vi "LevMar - abx.vi"(0 "Y":dbl[](array[numeric]) format="%0.2f", 1 "Target function in":refnum<vi>, 2 "Coefficients":dbl[](array[numeric]) format="%0.2f", 3 "Standard Deviation":dbl[](array[numeric]) caption="Écart-type" format="%0.2f") -> (5 "Target function out":refnum<vi>, 6 "Alpha":dbl[][](array[numeric]) format="%0.2f", 7 "Beta":dbl[](array[numeric]) caption="Bêta" format="%0.2f", 9 "chiSqr":dbl caption="khiCarré" format="%0.2f")   [LabVIEW 2009]
panel:
  # "Lev-Mar\nabx"
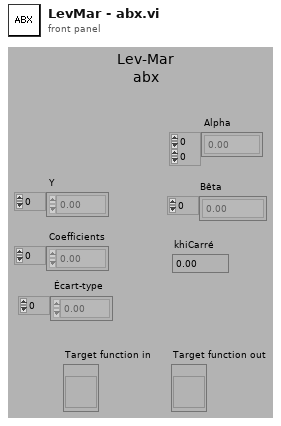
[diagram p1: front panel]
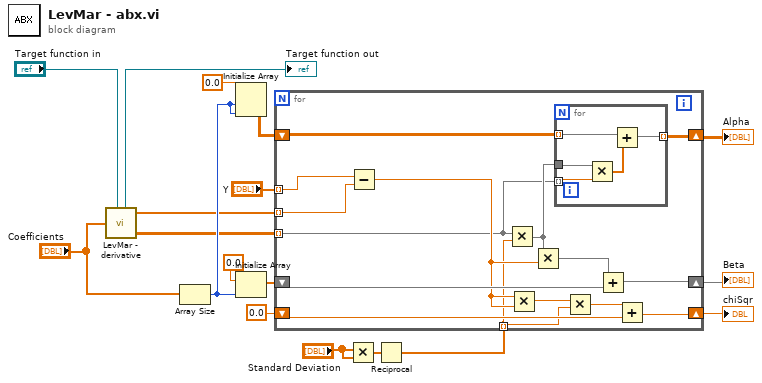
[diagram p0: block diagram]
diagram:
  n1 = call "LevMar - derivative.vi"("Target Function in"="Target function in", "Coefficients"="Coefficients") -> ("Target Function out"=→"Target function out":refnum<vi>, "F"=w2:dbl[], "dF/dA"=w4:dbl[][])  [unwired: 5 in]
  n2 = Array Size(array="Coefficients") -> (size(s)=w17:i32)
  n3 = Initialize Array(0.0, w17, w17) -> (w15:dbl[][])
  n4 = Initialize Array(0.0, w17) -> (w16:dbl[])
  n5 = Multiply(x="Standard Deviation", y="Standard Deviation") -> (x*y=w8:dbl[])
  n6 = Reciprocal(x=w8) -> (1/x=w6:dbl[])
  n7 = for {
    shift-right: [w29] -> w13
    shift-left: w16 -> [w30]
    shift-right: [w26] -> w10
    shift-left: w15 -> [w27]
    shift-right: [w25] -> w7
    shift-left: 0.0 -> [w32]
    tunnel: "Y" -> [w31] mode=indexing
    tunnel: w6 -> [w22] mode=indexing
    tunnel: w4 -> [w21] mode=indexing
    tunnel: w2 -> [w20] mode=indexing
    n8 = Subtract(x=w31, y=w20) -> (x-y=w28:dbl)
    n9 = Multiply(x=w21, y=w22) -> (x*y=w24:dbl[])
    n10 = Multiply(x=w28, y=w28) -> (x*y=w33:dbl)
    n11 = Multiply(x=w24, y=w28) -> (x*y=w19:dbl[])
    n12 = for {
      tunnel: w24 -> [w38]
      tunnel: w27 -> [w37] mode=indexing
      tunnel: [w36] -> w26 mode=indexing
      tunnel: w21 -> [w35] mode=indexing
      n13 = Multiply(x=w38, y=w35) -> (x*y=w34:dbl[])
      n14 = Add(x=w37, y=w34) -> (x+y=w36:dbl[])
    }
    n15 = Multiply(x=w33, y=w22) -> (x*y=w23:dbl)
    n16 = Add(x=w19, y=w30) -> (x+y=w29:dbl[])
    n17 = Add(x=w23, y=w32) -> (x+y=w25:dbl)
  }
  "Alpha" <- w10
  "Beta" <- w13
  "chiSqr" <- w7
